vi "未初始化移位寄存器.vi"() -> ()   [LabVIEW 2020]
doc: "本VI是为《我和LabVIEW》一书编写的示例。\n关于本书的介绍请参考网页：\nhttp://ruanqizhen.spaces.live.com/blog/cns!5852D4F797C53FB6!4310.entry"
panel:
  out "输出值 2":i32
  out "输出值":i32
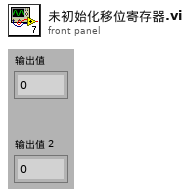
[diagram p1: front panel]
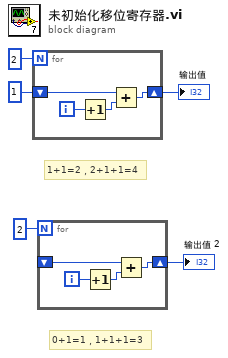
[diagram p0: block diagram]
diagram:
  # "0+1=1，1+1+1=3"
  # "1+1=2，2+1+1=4"
  n1 = for {
    N: 2 -> [_]
    shift-right: [w7] -> w5
    shift-left: 1 -> [w9]
    i -> [w8]
    n2 = Increment(x=w8) -> (x+1=w6:i32)
    n3 = Add(x=w9, y=w6) -> (x+y=w7:i32)
  }
  "输出值" <- w5
  n4 = for {
    N: 2 -> [_]
    shift-right: [w11] -> w2
    shift-left: _ -> [w13]
    i -> [w12]
    n5 = Increment(x=w12) -> (x+1=w10:i32)
    n6 = Add(x=w13, y=w10) -> (x+y=w11:i32)
  }
  "输出值 2" <- w2
